vi "visa tool.vi"(8 "error in (no error)":errorcluster, 9 "Opciones":T1(ring), 10 "Write":string, 11 "VISA com port":refnum<visa-resource-name>) -> (0 "error out":errorcluster, 1 "Read":string, 3 "VISA com port 2":refnum<visa-resource-name>)   [LabVIEW 2020]
uses:
  <vilib>/Instr/_visa.llb/VISA Configure Serial Port (Instr).vi
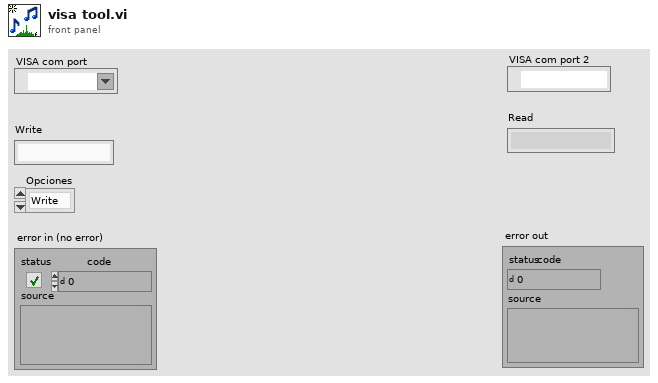
[diagram p1: front panel]
types:
  T1 = enum16{"Write", "Read", "Config", "Reset", "Close"}
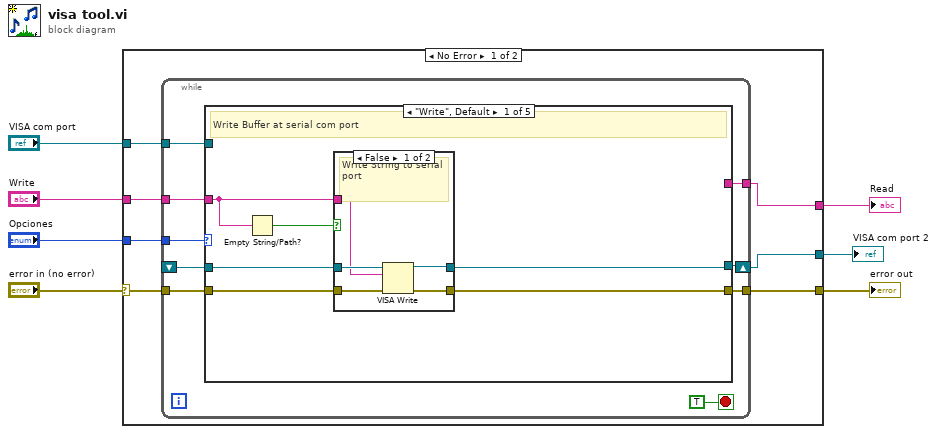
[diagram p0: block diagram]
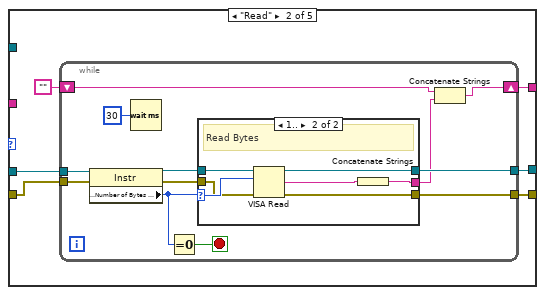
[diagram p3: hidden frame]
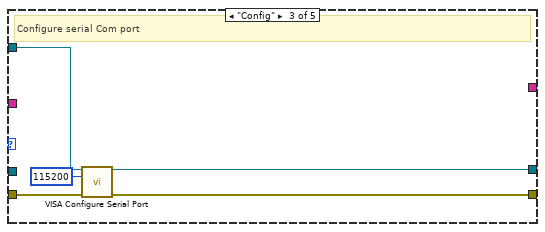
[diagram p5: hidden frame]
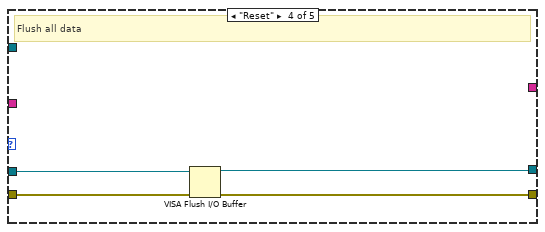
[diagram p6: hidden frame]
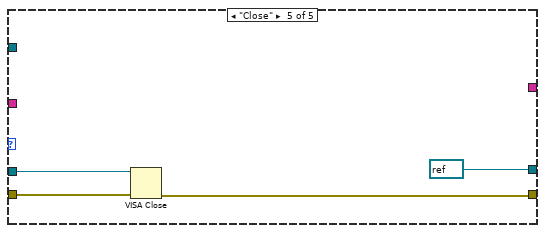
[diagram p7: hidden frame]
diagram:
  n1 = case shown="No Error" "error in (no error)" {
    selector: "error in (no error)" -> [w13 w77]
    tunnel: [w12 w77] -> w6
    tunnel: "Opciones" -> [w14 _]
    tunnel: "VISA com port" -> [w11 _]
    tunnel: "Write" -> [w10 _]
    tunnel: [w9 _] -> w2
    tunnel: [w8 _] -> w1
    frame No Error {
      n2 = while {
        tunnel: w14 -> [w22]
        tunnel: w13 -> [w21]
        tunnel: [w20] -> w12
        tunnel: w11 -> [w19]
        shift-right: [w18] -> w8
        shift-left: _ -> [w17]
        tunnel: w10 -> [w16]
        tunnel: [w15] -> w9
        stop <- TRUE stop-if-true
        n3 = case shown="\"Write\", Default" w22 {
          tunnel: w21 -> [w29 w41 w68 w72 w76]
          tunnel: [w28 w40 w64 w71 w75] -> w20
          tunnel: w19 -> [_ _ w67 _ _]
          tunnel: [w24 w39 w66 w69 refnum<visa-resource-name> refnum ("VISA resource name out")] -> w18
          tunnel: w17 -> [w27 w42 _ w70 w74]
          tunnel: w16 -> [w26 _ _ _ _]
          tunnel: [_ w38 _ _ _] -> w15
          frame "Write", Default {
            # "Write Buffer at serial com port"
            n4 = Empty String/Path?(string/path=w26) -> (empty?=w25:bool)
            n5 = case shown="False" w25 {
              tunnel: w29 -> [w34 w35]
              tunnel: [w33 w35] -> w28
              tunnel: w27 -> [w32 w36]
              tunnel: w26 -> [w31 _]
              tunnel: [w30 w36] -> w24
              frame False {
                # "Write String to serial port"
                n6 = VISA Write(VISA resource name=w32, write buffer=w31, error in (no error)=w34) -> (VISA resource name out=w30:refnum<visa-resource-name>, error out=w33:errorcluster)  [unwired: 1 out]
              }
              frame True {
              }
            }
          }
          frame "Read" {
            n7 = while {
              tunnel: w42 -> [w54]
              tunnel: w41 -> [w53]
              tunnel: [w50] -> w40
              tunnel: [w49] -> w39
              shift-right: [w44] -> w38
              shift-left: "" -> [w43]
              stop <- w46 stop-if-true
              n8 = property class="Instr"(reference=w54, error in=w53) -> (reference out=w52:refnum<visa-resource-name>, error out=w51:errorcluster, "Serial Settings:Number of Bytes at Serial Port"=w47:u32)
              n9 = Wait (ms)(milliseconds to wait=u32 30) -> ()  [unwired: 1 out]
              n10 = Equal To 0?(x=w47) -> (x = 0?=w46:bool)
              n11 = case shown="1.." w47 {
                selector: w47 -> [_ w62]
                tunnel: w52 -> [w56 w63]
                tunnel: w51 -> [w55 w59]
                tunnel: [w55 w61] -> w50
                tunnel: [w56 w60] -> w49
                tunnel: [_ w57] -> w45
                frame 0, Default {
                }
                frame 1.. {
                  # "Read Bytes"
                  n12 = VISA Read(VISA resource name=w63, byte count=w62, error in (no error)=w59) -> (VISA resource name out=w60:refnum<visa-resource-name>, read buffer=w58:string, error out=w61:errorcluster)  [unwired: 1 out]
                  n13 = Concatenate Strings(w58) -> (w57:string)
                }
              }
              n14 = Concatenate Strings(w43, w45) -> (w44:string)
            }
          }
          frame "Config" {
            # "Configure serial Com port"
            n15 = call-poly "VISA Configure Serial Port"("VISA resource name"=w67, "baud rate (9600)"=u32 115200, "error in (no error)"=w68) -> ("VISA resource name out"=w66:refnum<visa-resource-name>, "error out"=w64:errorcluster)  [unwired: 11 in]
          }
          frame "Reset" {
            # "Flush all data"
            n16 = VISA Flush I/O Buffer(VISA resource name=w70, error in (no error)=w72) -> (VISA resource name out=w69:refnum<visa-resource-name>, error out=w71:errorcluster)  [unwired: 1 in]
          }
          frame "Close" {
            n17 = VISA Close(VISA resource name=w74, error in (no error)=w76) -> (error out=w75:errorcluster)
          }
        }
      }
    }
    frame Error {
    }
  }
  "error out" <- w6
  "Read" <- w2
  "VISA com port 2" <- w1
